vi "DHE_DRV_set_cont_read.vi"(8 "error in (no error)":errorcluster, 10 "arg1":i32, 11 "fd":i32) -> (0 "error out":errorcluster, 2 "error_code":i32, 3 "fd":i32)   [LabVIEW 2016]
doc: "This VI closes the I/O interface with the instrument."
uses:
  c/lib/libarcDHE.so
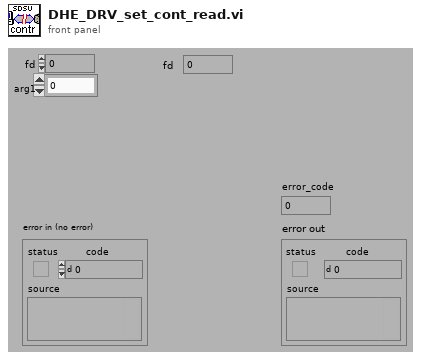
[diagram p1: front panel]
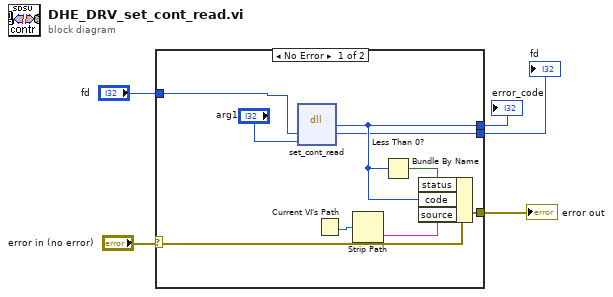
[diagram p0: block diagram]
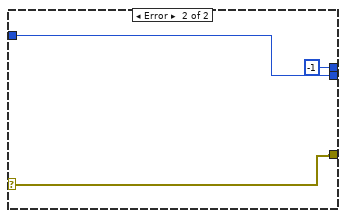
[diagram p2: hidden frame]
diagram:
  n1 = case shown="No Error" "error in (no error)" {
    selector: "error in (no error)" -> [w8 w17]
    tunnel: [w13 -1] -> w5
    tunnel: [w10 w17] -> w4
    tunnel: [w9 w16] -> w3
    tunnel: "fd" -> [w7 w16]
    frame No Error {
      n2 = dll-call lib="home/simager/panview/PAN/Modules/SDSU/private/c/lib/libarcDHE.so" fn="set_cont_read" label="cont_read"("fd"=w7, "cont_read"="arg1") -> (w13:i32, "fd"=w9:i32)  [unwired: 4 in, 2 out]
      n3 = Current VI's Path() -> (path=w12:path)
      n4 = Strip Path(path=w12) -> (name=w11:string)  [unwired: 1 out]
      n5 = Less Than 0?(x=w13) -> (x < 0?=w14:bool)
      n6 = Bundle By Name(cluster=w8, "status"=w14, "code"=w13, "source"=w11) -> (w10:errorcluster)
    }
    frame Error {
    }
  }
  "error out" <- w4
  "error_code" <- w5
  "fd" <- w3
